vi "P2018 TB INCAR_Initialize.vi"(8 "error in (no error)":errorcluster, 11 "User event":T4) -> (0 "error out":errorcluster, 1 "MassFlow":T1={"Dispositivos"=[["3", "NO", "M0000013", "Air", "10", "ln/mn", "0", "0"], ["4", "NO", "M0000014", "Air", "10", "ln/mn", "0", "0"], ["5", "NO", "M0000015", "Air", "10", "ln/mn", "0", "0"], ["6", "NO", "M0000016", "Air", "10", "ln/mn", "0", "0"], ["7", "NO", "M0000017", "Air", "10", "ln/mn", "0", "0"], ["8", "NO", "M0000018", "Air", "10", "ln/mn", "0", "0"]], "NuevosSP"=[["0", "NO", "M0000013", "Air", "1", "ln/mn", "0", "0"], ["0", "NO", "M0000014", "Air", "1", "ln/mn", "0", "0"], ["0", "NO", "M0000015", "Air", "1", "ln/mn", "0", "0"], ["0", "NO", "M0000016", "Air", "1", "ln/mn", "0", "0"], ["0", "NO", "M0000017", "Air", "1", "ln/mn", "0", "0"], ["0", "NO", "M0000018", "Air", "1", "ln/mn", "0", "0"]], "Nodes"=4, "Delay(s)"=0.075}, 3 "Comunicaciones":T3={"Flujo_1"="ASRL6::INSTR", "Brk1"=FALSE, "Flujo_2"="ASRL6::INSTR", "Brk2"=FALSE, "Flujo_3"="ASRL6::INSTR", "Brk3"=FALSE, "Flujo_4"="ASRL6::INSTR", "Brk4"=FALSE, "Eurothe"="ASRL6::INSTR", "Eurot"=FALSE, "Balanza"="ASRL6::INSTR", "Bal"=FALSE, "eValPos"="ASRL6::INSTR", "eVal"=FALSE, "flowbus"="ASRL6::INSTR", "fb"=FALSE})   [LabVIEW 2013]
uses:
  Display/Display_Command Control.ctl
  Controles/Data Type.ctl
  serialTermobDisbal/Multicard III_Hardware_Module Control.ctl
  serialArduinoMicro/ArduinoMicro Module Control.ctl
  modbusEurotherm P116_485/Eurotherm_Hardware_Module Control.ctl
  P2022 TB INCAR GLOBALES.vi
  serialBronkhorst/_s_TablaBronkhorst.ctl
  Controles/P2018 Bronkhorst Control.ctl
  Controles/User Event Data.ctl
  Controles/User Event Reference.ctl
  Controles/P2018 Com Control.ctl
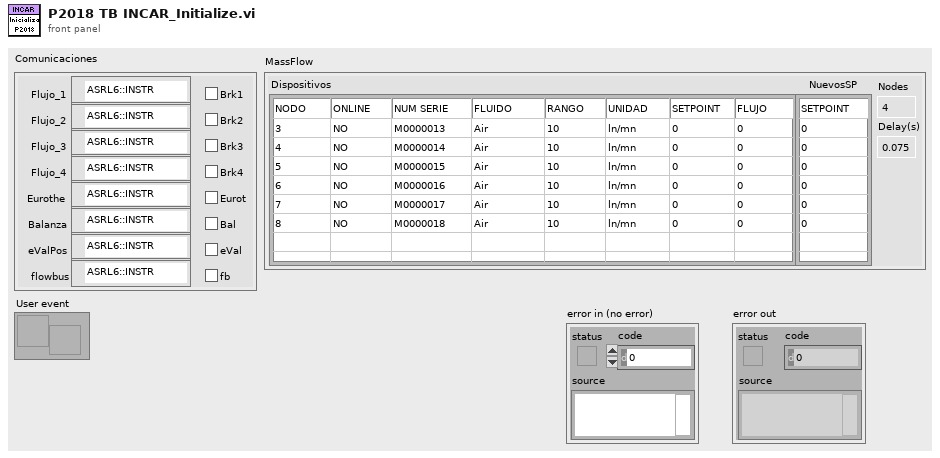
[diagram p1: front panel]
types:
  T1 = typedef "P2018 Bronkhorst Control.ctl" = cluster{"Dispositivos":T2, "NuevosSP":string[][], "Nodes":u32, "Delay(s)":dbl}
  T2 = typedef "_s_TablaBronkhorst.ctl" = string[][]
  T3 = typedef "P2018 Com Control.ctl" = cluster{"Flujo_1":refnum<visa-resource-name>, "Brk1":bool, "Flujo_2":refnum<visa-resource-name>, "Brk2":bool, "Flujo_3":refnum<visa-resource-name>, "Brk3":bool, "Flujo_4":refnum<visa-resource-name>, "Brk4":bool, "Eurothe":refnum<visa-resource-name>, "Eurot":bool, "Balanza":refnum<visa-resource-name>, "Bal":bool, "eValPos":refnum<visa-resource-name>, "eVal":bool, "flowbus":refnum<visa-resource-name>, "fb":bool}
  T4 = typedef "User Event Reference.ctl" = refnum<user-event>
  T5 = typedef "ArduinoMicro Module Control.ctl" = enum16{"Initialize", "Read Data", "Write Data", "Enable", "Disable", "Shutdown"}
  T6 = typedef "Multicard III_Hardware_Module Control.ctl" = enum16{"Initialize", "Cero", "Span", "Read ugr", "Read mgr", "Read A/D", "Read T", "Number readings", "Thermocouple type", "Status", "Shutdown"}
  T7 = typedef "Data Type.ctl" = enum16{"Init FP", "En/Dis FP Ctls", "Update FP", "Upd Status", "Upd Seq"}
  T8 = typedef "Display_Command Control.ctl" = enum16{"Initialize", "Generate Event", "Shutdown"}
  T9 = typedef "Eurotherm_Hardware_Module Control.ctl" = enum16{"Initialize", "Write SP", "Read SP+PV", "Write Rate", "Set P", "Set I", "Set D", "Shutdown"}
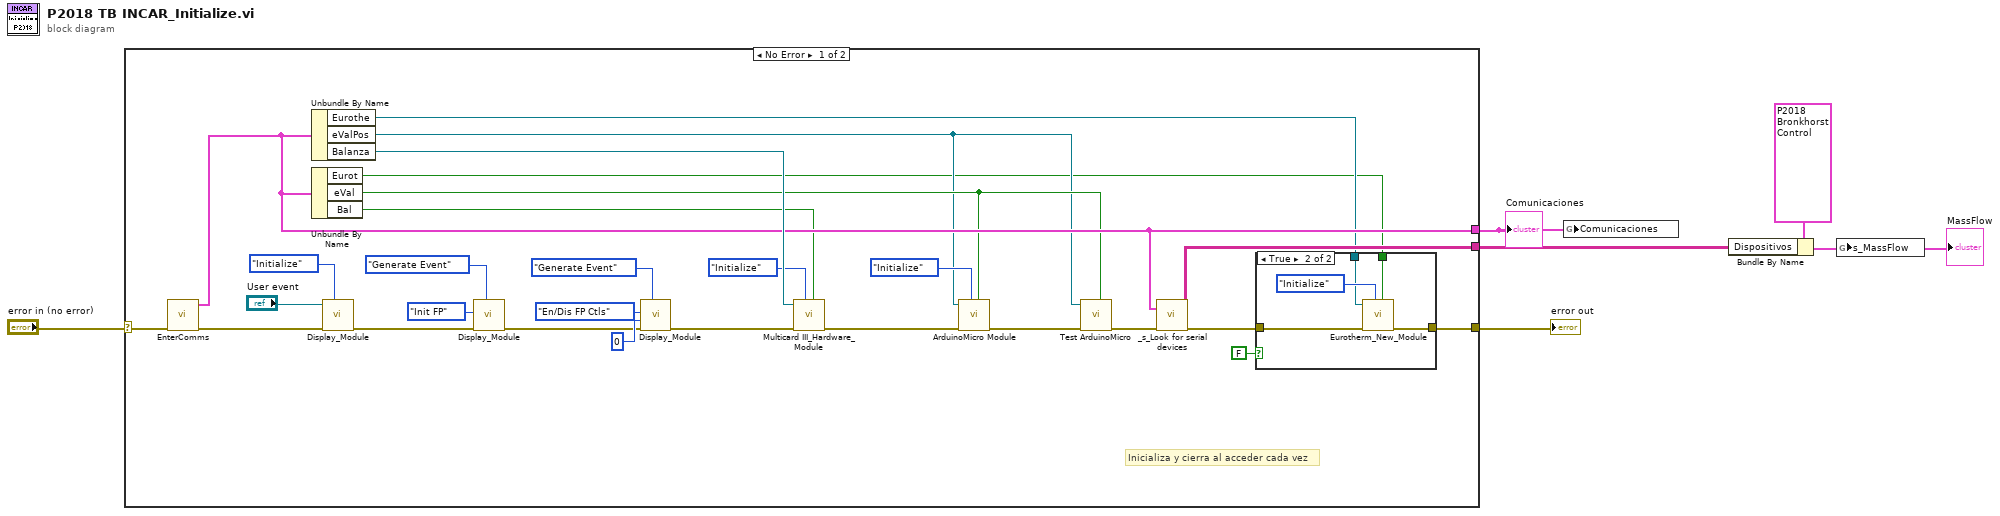
[diagram p0: block diagram]
diagram:
  n1 = case shown="No Error" "error in (no error)" {
    selector: "error in (no error)" -> [w30 w41]
    tunnel: [w11 w41] -> w5
    tunnel: [w15 _] -> w2
    tunnel: [w20 _] -> w3
    frame No Error {
      # "Inicializa y cierra al acceder cada vez"
      n2 = call "EnterComms.vi"("error in (no error)"=w30) -> ("error out"=w19:errorcluster, "Comunicaciones"=w15:T3)  [unwired: 8 in, 1 out]
      n3 = Unbundle By Name(w15) -> ("Eurothe"=w10:refnum<visa-resource-name>, "eValPos"=w13:refnum<visa-resource-name>, "Balanza"=w24:refnum<visa-resource-name>)
      n4 = Unbundle By Name(w15) -> ("Eurot"=w9:bool, "eVal"=w14:bool, "Bal"=w8:bool)
      n5 = call "Display_Module.vi"("Command"=Display_Command_Control."Initialize", "error in (no error)"=w19, "user event out"="User event") -> ("error out"=w32:errorcluster)  [unwired: 8 in]
      n6 = call "Display_Module.vi"("Command"=Display_Command_Control."Generate Event", "error in (no error)"=w32, "Data Type"=Data_Type."Init FP") -> ("error out"=w31:errorcluster)  [unwired: 8 in]
      n7 = call "Display_Module.vi"("Command"=Display_Command_Control."Generate Event", "error in (no error)"=w31, "Data"=0, "Data Type"=Data_Type."En/Dis FP Ctls") -> ("error out"=w16:errorcluster)  [unwired: 7 in]
      n8 = call "Multicard III_Hardware_Module.vi"("Multicard (T:Enable)"=w8, "Command"=Multicard_III_Hardware_Module_Control."Initialize", "error in (no error)"=w16, "VISA resource name"=w24) -> ("error out"=w21:errorcluster)  [unwired: 4 in, 3 out]
      n9 = call "ArduinoMicro Module.vi"("Enable"=w14, "Command"=ArduinoMicro_Module_Control."Initialize", "error in (no error)"=w21, "VISA resource name"=w13) -> ("error out"=w18:errorcluster)  [unwired: 3 in, 4 out]
      n10 = call "Test ArduinoMicro.vi"("Enable"=w14, "error in"=w18, "VISA resource name"=w13) -> ("error out"=w17:errorcluster)  [unwired: 8 in]
      n11 = call "_s_Look for serial devices.vi"("Comunicaciones"=w15, "error in (no error)"=w17) -> ("error out"=w12:errorcluster, "Dispositivos"=w20:T2)  [unwired: 8 in]
      n12 = case shown="True" FALSE {
        tunnel: w12 -> [w35 w40]
        tunnel: [w35 w39] -> w11
        tunnel: w10 -> [_ w37]
        tunnel: w9 -> [_ w36]
        frame False {
        }
        frame True {
          n13 = call "Eurotherm_New_Module.vi"("Eurotherm (T:Enable)"=w36, "Command"=Eurotherm_Hardware_Module_Control."Initialize", "error in (no error)"=w40, "VISA resource name"=w37) -> ("error out"=w39:errorcluster)  [unwired: 6 in, 1 out]
        }
      }
    }
    frame Error {
    }
  }
  "error out" <- w5
  "Comunicaciones" <- w2
  n14 = global write "P2022 TB INCAR GLOBALES.vi" "Comunicaciones"(w2) -> ()
  n15 = Bundle By Name(cluster=T1 {"Dispositivos"=[["3", "NO", "M0000013", "Air", "10", "ln/mn", "0", "0"], ["4", "NO", "M0000014", "Air", "10", "ln/mn", "0", "0"], ["5", "NO", "M0000015", "Air", "10", "ln/mn", "0", "0"], ["6", "NO", "M0000016", "Air", "10", "ln/mn", "0", "0"], ["7", "NO", "M0000017", "Air", "10", "ln/mn", "0", "0"], ["8", "NO", "M0000018", "Air", "10", "ln/mn", "0", "0"]], "NuevosSP"=[["0", "NO", "M0000013", "Air", "1", "ln/mn", "0", "0"], ["0", "NO", "M0000014", "Air", "1", "ln/mn", "0", "0"], ["0", "NO", "M0000015", "Air", "1", "ln/mn", "0", "0"], ["0", "NO", "M0000016", "Air", "1", "ln/mn", "0", "0"], ["0", "NO", "M0000017", "Air", "1", "ln/mn", "0", "0"], ["0", "NO", "M0000018", "Air", "1", "ln/mn", "0", "0"]], "Nodes"=4, "Delay(s)"=0.075} ("MassFlow"), "Dispositivos"=w3) -> (w1:T1)
  "MassFlow" <- w1
  n16 = global write "P2022 TB INCAR GLOBALES.vi" "s_MassFlow"(w1) -> ()
